vi "set_cal_info.vi"(6 "timeout (25000ms)":i32=25000, 8 "error in (no error)":errorcluster, 9 "Parameter":T2, 10 "Mode":T1, 11 "daemon reference in":refnum<k5>) -> (0 "error out":errorcluster, 2 "response":string, 3 "daemon reference out":refnum<k5>, 5 "command out":string="random")   [LabVIEW 2017]
doc: "<b>Command: </b>\"set_cal_info\"\n\n<b>Description: </b> This command request device to write FCT/EOL/PROD calibration information. \n\n<b>Parameters: </b> Mode, Timestamp, Rig ID , Passmark ID , Passmark Revision\n____________________________________________\nDIPC 692 Daemon API 10.0.0.1\nSam Tee - Dyson Technology Ltd\nCopyright (c) 2024, Dyson Technology Ltd"
uses:
  typdef/device_mode.ctl
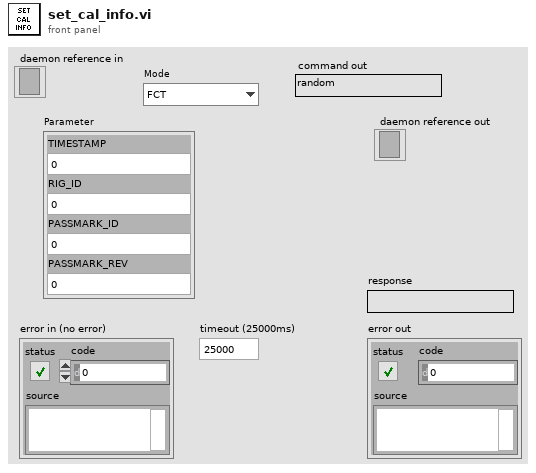
[diagram p1: front panel]
types:
  T1 = typedef "device_mode.ctl" = enum16{"FCT", "EOL", "PROD"}
  T2 = cluster{"TIMESTAMP":i64, "RIG_ID":i64, "PASSMARK_ID":i64, "PASSMARK_REV":i64}
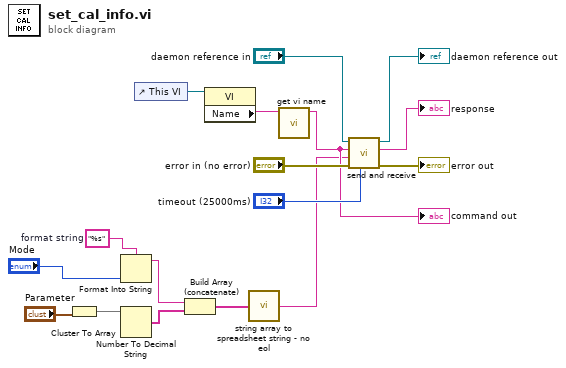
[diagram p0: block diagram]
diagram:
  w3 = "%s"  # format string
  n1 = Cluster To Array(cluster="Parameter") -> (array=w7:i64[])
  n2 = Format Into String(format string=w3, "Mode") -> (resulting string=w1:string)  [unwired: 2 in, 1 out]
  n3 = Number To Decimal String(number=w7) -> (decimal integer string=w5:string[])  [unwired: 1 in]
  n4 = control-ref of="This VI"() -> (w11:refnum<vi>)
  n5 = Build Array (concatenate)(w1, w5) -> (w4:string[])
  n6 = property class="VI"(reference=w11) -> ("Name"=w10:string)  [unwired: 1 in, 2 out]
  n7 = call "string array to spreadsheet string - no eol.vi"("string array"=w4) -> ("spreadsheet string - no eol"=w6:string)
  n8 = call "get vi name.vi"("library.lvlib:name.vi"=w10) -> ("vi name"=w9:string)  [unwired: 10 in]
  "command out" <- w9
  n9 = call "send and receive.vi"("timeout (25000ms)"="timeout (25000ms)", "error in (no error)"="error in (no error)", "data"=w6, "command"=w9, "daemon reference in"="daemon reference in") -> ("error out"=→"error out":errorcluster, "response"=→"response":string, "daemon reference out"=→"daemon reference out":refnum<k5>)  [unwired: 4 in]
